vi "Mapping v10.6.4.vi"(5 "Simulate Spectra":bool, 7 "Simulate Drive":bool) -> ()   [LabVIEW 2010]
uses:
  TypeDefs/Mapping Spectra Params.ctl
  TypeDefs/Mapping Drive Params v10.6.0.ctl
  NPC3SG/TypeDefs/NPC3SG Set Positions.ctl
  NPC3SG/TypeDefs/NPC3SG Current Values.ctl
  iHR550/TypeDefs/iHR Current Values.ctl
  ITC503/TypeDefs/ITC503 Current Values.ctl
  TypeDefs/Mapping Input Parameters v10.6.2.ctl
  Symphony/TypeDefs/Symphony Area Format.ctl
  <vilib>/Utility/miscctls.llb/LVPointTypeDef.ctl
  Global Variables.vi
panel:
  in  "AutoSave Inc.":i16=20 caption="Auto Save (%)" min=10 max=160 step=1
  in  "Save Map":bool
  in  "Input Parameters":T1={"Drive Connection Port"="", "ITC503 Current Values"={"ITC503 Heater"=0.0, "ITC503 Temperature"=0.0, "ITC503 P"=0.0, "ITC503 I"=0.0, "ITC503 D"=0.0, "ITC503 Setpoint"=0.0, "ITC503 Gradient"=0.0, "ITC503 Heater Auto"=FALSE, "ITC503 PID Auto"=FALSE}, "Wavelengths (nm)"=[], "Drive Current Values"={"Drive X Position"=0.0, "Drive Y Position"=0.0, "Drive Z Position"=0.0}, "iHR Current Values"={"iHR 550 Front Entrance"=0.0, "iHR550 Side Exit"=0.0, "iHR550 Wavelength"=897.9988, "iHR550 Exit Mirror"=2, "iHR550 Grating"="1", "Grating Index"=1}, "Spectra Settings"={"Integration Time"=1.0, "Repetitions"=1, "Mapping Spectra"=TRUE}, "CCD3500 Temperature"=0.0, "Simulate Drive"=FALSE, "Simulate Spectra"=FALSE, "JYCCDLib.IJYCCDReqd"=refnum, "CCD Area"={"XStart"=1, "YStart"=1, "XStop"=2048, "YStop"=512, "XBin"=1, "YBin"=1}, "CCD Gain"=1, "CCD ADC"=0, "Drive Calibration"=path ""} {"CCD ADC" items=["20 kHz       ", " 1 MHz       ", " 1 MHz Ultra ", "500 kHz Wrap"]; "CCD Gain" items=["High Light", "Best Dynamic Range", "High Sensitivity"]; "ITC503 Current Values"."ITC503 Gradient" format="%.2f"; "ITC503 Current Values"."ITC503 Setpoint" min=-273.0 max=300000.0 step=0.0001 format="%.1f"; "ITC503 Current Values"."ITC503 I" format="%_1f"; "ITC503 Current Values"."ITC503 P" format="%_1f"; "ITC503 Current Values"."ITC503 Temperature" min=0.0 max=1645.0 step=1e-05 format="%.2f"; "ITC503 Current Values"."ITC503 Heater" min=0.0 max=100.0 step=0.01 scale=0.0..100.0; "Drive Current Values"."Drive Z Position" min=-273.0 max=300000.0 step=0.0001 format="%.3f"; "Drive Current Values"."Drive Y Position" min=-273.0 max=300000.0 step=0.0001 format="%.3f"; "Drive Current Values"."Drive X Position" min=-273.0 max=300000.0 step=0.0001 format="%.3f"; "iHR Current Values"."iHR550 Exit Mirror" items=["EntranceMirror", "ExitMirror", "Front", "Side"]; "Spectra Settings"."Repetitions" min=1 max=100 step=1; "Spectra Settings"."Integration Time" min=0.5 max=6000.0 step=1.0 format="%.1f"}
  out "JYCCDLib.IJYCCDReqd":refnum<k7>
  out "AutoClose":bool
  out "ITC503 Temperature":dbl caption="Sample (K)" min=10.0 max=160.0 step=0.1 format="%.3f"
  out "CCD3500 Temperature":dbl caption="CCD (°C)" min=10.0 max=160.0 step=0.1 format="%.1f"
  in  "CCD Current Rep.":string="0/0"
  in  "Pause":bool
  out "Current Position":T3 {"Drive Z Position" min=-273.0 max=300000.0 step=0.0001 format="%.3f"; "Drive Y Position" min=-273.0 max=300000.0 step=0.0001 format="%.3f"; "Drive X Position" min=-273.0 max=300000.0 step=0.0001 format="%.3f"}
  out "Target Position":T7={"Drive X Set"=10.0, "Drive Y Set"=10.0, "Drive Z Set"=10.0} {"Drive X Set" min=10.0 max=160.0 step=0.1 format="%.3f"; "Drive Z Set" min=10.0 max=160.0 step=0.1 format="%.3f"; "Drive Y Set" min=10.0 max=160.0 step=0.1 format="%.3f"}
  out "Progress":u8(slide) max=10 scale=0.0..100.0
  out "Objective Running":bool caption="Obj."
  out "CCD Running":bool caption="CCD"
  in  "Spectra Params":T5={"Integration Time"=10.0, "Repetitions"=10, "Mapping Spectra"=TRUE} {"Repetitions" min=1 max=100 step=1; "Integration Time" min=0.5 max=6000.0 step=1.0 format="%.1f"}
  in  "Drive Settings":refnum<visa-resource-name>
  in  "Z Position":dbl caption="Z (µm)" min=0.0 max=100.0 step=0.1 format="%.1f"
  in  "Mapping Params":T8={"X Start Position"=0.0, "X Stop Position"=10.0, "Y Start Position"=0.0, "Y Stop Position"=10.0, "Step Size"=1.0} {"Step Size" min=0.005 max=20.0 step=0.005 format="%.3f"; "Y Stop Position" min=0.0 max=140.0 step=0.005 format="%.3f"; "Y Start Position" min=0.0 max=140.0 step=0.005 format="%.3f"; "X Stop Position" min=0.0 max=140.0 step=0.005 format="%.3f"; "X Start Position" min=0.0 max=140.0 step=0.005 format="%.3f"}
  in  "Exit":bool
  out "Measuring":bool
  in  "Start":bool
  out "Filename":string
  out "Full Data":dbl[][](array[numeric])
  out "Live Data":dbl[][](array[numeric])
  in  "ITC503 Current Values":T2 {"ITC503 Gradient" format="%.2f"; "ITC503 Setpoint" min=-273.0 max=300000.0 step=0.0001 format="%.1f"; "ITC503 I" format="%_1f"; "ITC503 P" format="%_1f"; "ITC503 Temperature" min=0.0 max=1645.0 step=1e-05 format="%.2f"; "ITC503 Heater" min=0.0 max=100.0 step=0.01 scale=0.0..100.0}
  in  "iHR Current Values":T4={"iHR 550 Front Entrance"=0.0, "iHR550 Side Exit"=0.0, "iHR550 Wavelength"=897.9988, "iHR550 Exit Mirror"=2, "iHR550 Grating"="1", "Grating Index"=1} {"iHR550 Exit Mirror" items=["EntranceMirror", "ExitMirror", "Front", "Side"]}
  in  "Wavelengths (nm)":dbl[](array[numeric])
  # "Mapping"
  # "Status"
  # "Active"
  # "Target"
  # "Current"
  # "Spectral"
  # "Spectral / Video Mapping"
  # "Drive Settings"
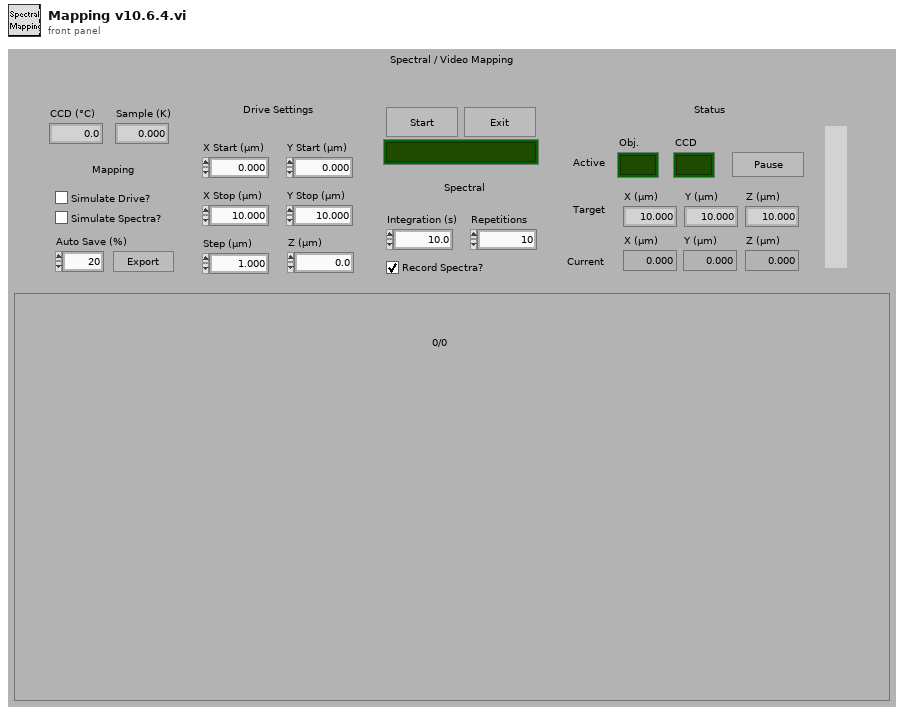
[diagram p1: front panel]
types:
  T1 = typedef "Mapping Input Parameters v10.6.2.ctl" = cluster{"Drive Connection Port":refnum<visa-resource-name>, "ITC503 Current Values":T2, "Wavelengths (nm)":dbl[], "Drive Current Values":T3, "iHR Current Values":T4, "Spectra Settings":T5, "CCD3500 Temperature":dbl, "Simulate Drive":bool, "Simulate Spectra":bool, "JYCCDLib.IJYCCDReqd":refnum<k7>, "CCD Area":T6, "CCD Gain":u16, "CCD ADC":u16, "Drive Calibration":path}
  T2 = typedef "ITC503 Current Values.ctl" = cluster{"ITC503 Heater":dbl, "ITC503 Temperature":dbl, "ITC503 P":dbl, "ITC503 I":dbl, "ITC503 D":dbl, "ITC503 Setpoint":dbl, "ITC503 Gradient":dbl, "ITC503 Heater Auto":bool, "ITC503 PID Auto":bool}
  T3 = typedef "NPC3SG Current Values.ctl" = cluster{"Drive X Position":dbl, "Drive Y Position":dbl, "Drive Z Position":dbl}
  T4 = typedef "iHR Current Values.ctl" = cluster{"iHR 550 Front Entrance":dbl, "iHR550 Side Exit":dbl, "iHR550 Wavelength":dbl, "iHR550 Exit Mirror":i32, "iHR550 Grating":string, "Grating Index":i32}
  T5 = typedef "Mapping Spectra Params.ctl" = cluster{"Integration Time":dbl, "Repetitions":u16, "Mapping Spectra":bool}
  T6 = typedef "Symphony Area Format.ctl" = cluster{"XStart":i32, "YStart":i32, "XStop":i32, "YStop":i32, "XBin":i32, "YBin":i32}
  T7 = typedef "NPC3SG Set Positions.ctl" = cluster{"Drive X Set":dbl, "Drive Y Set":dbl, "Drive Z Set":dbl}
  T8 = typedef "Mapping Drive Params v10.6.0.ctl" = cluster{"X Start Position":dbl, "X Stop Position":dbl, "Y Start Position":dbl, "Y Stop Position":dbl, "Step Size":dbl}
  T9 = typedef "LVPointTypeDef.ctl" = cluster{"Horizontal":i16, "Vertical":i16}
  T10 = cluster{"Intensities":dbl[], "Wavelengths":dbl[]}[]
  T11 = cluster{"Intensities":dbl[], "Wavelengths":dbl[]}
  T12 = enum32{"invalid app kind", "Development System", "Run Time System", "Student Edition", "Embedded LabVIEW", "Evaluation", "Custom"}
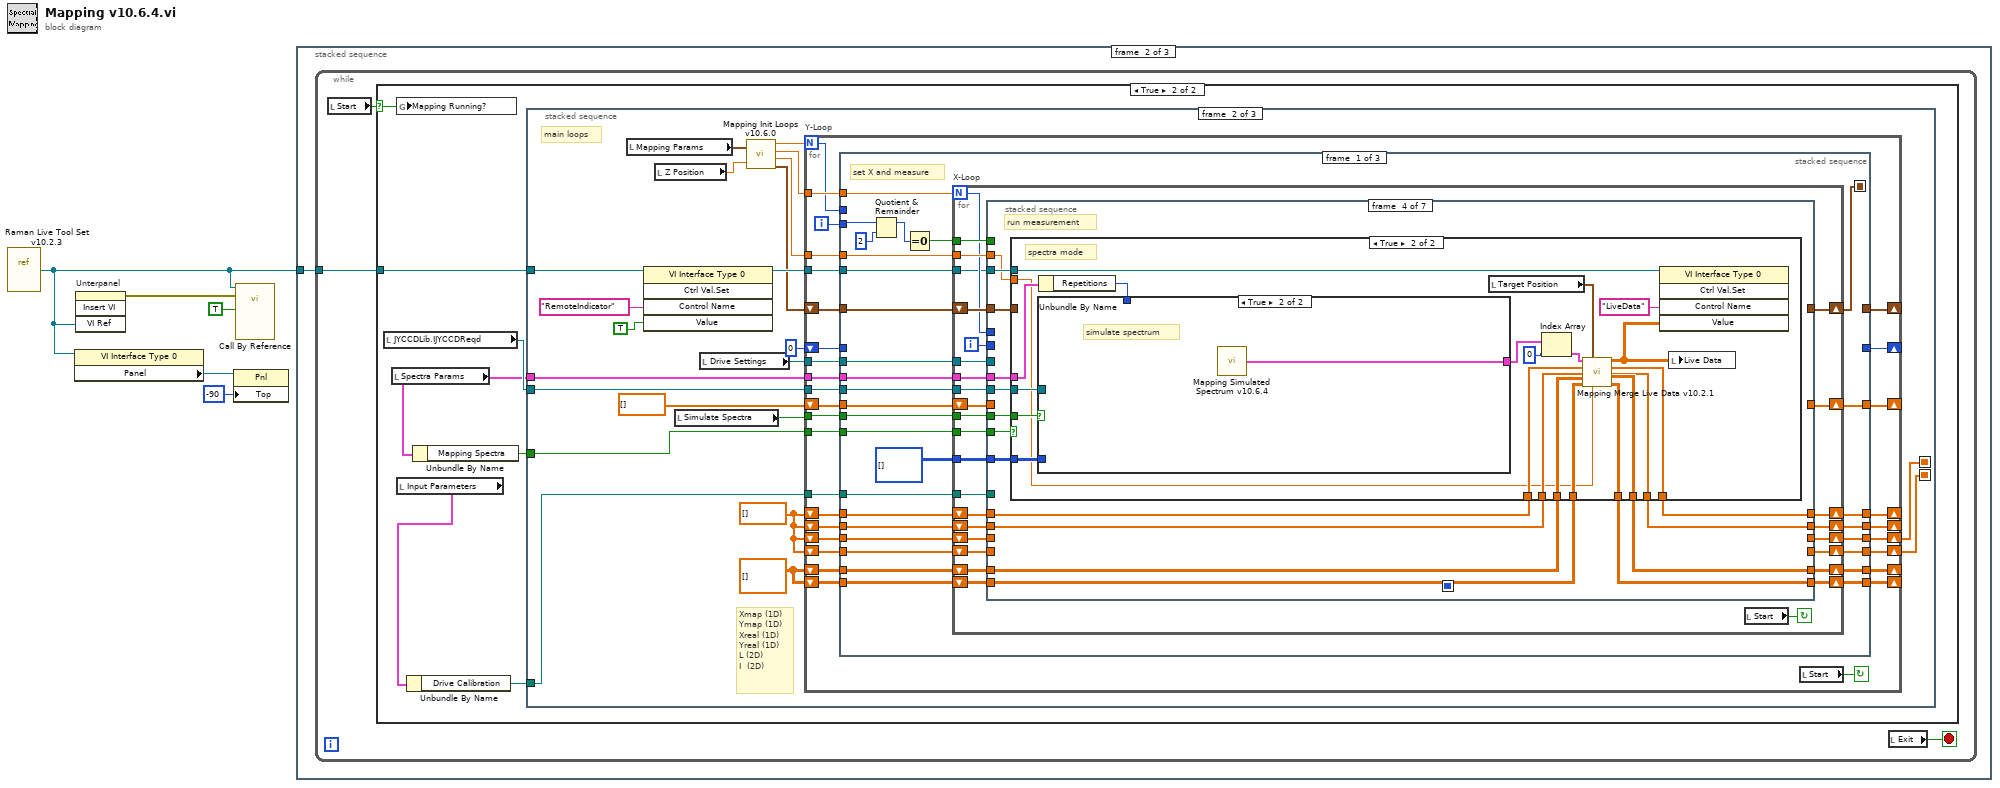
[diagram p0: block diagram]
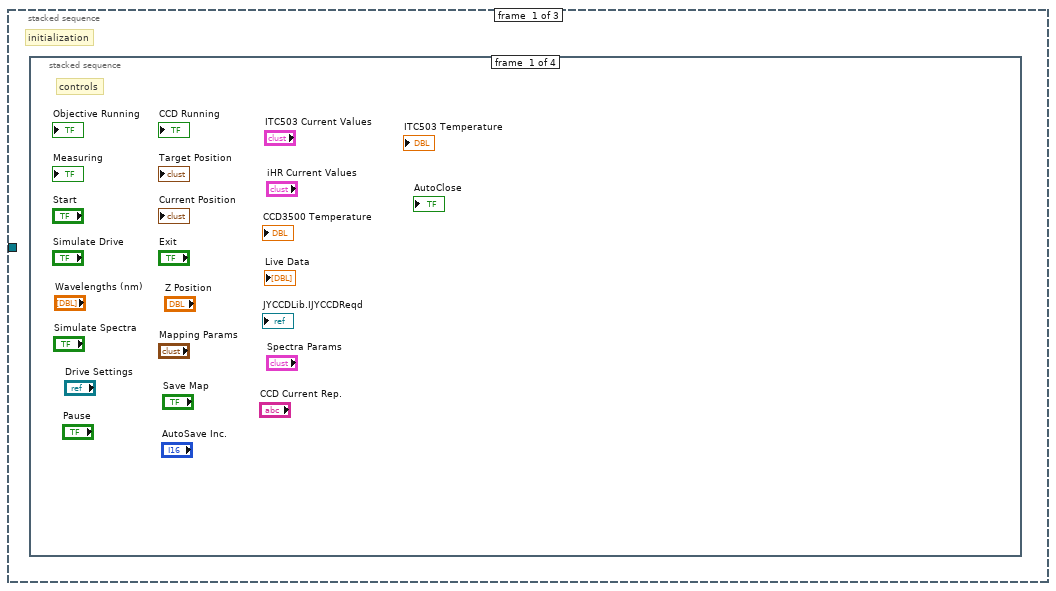
[diagram p2: hidden frame]
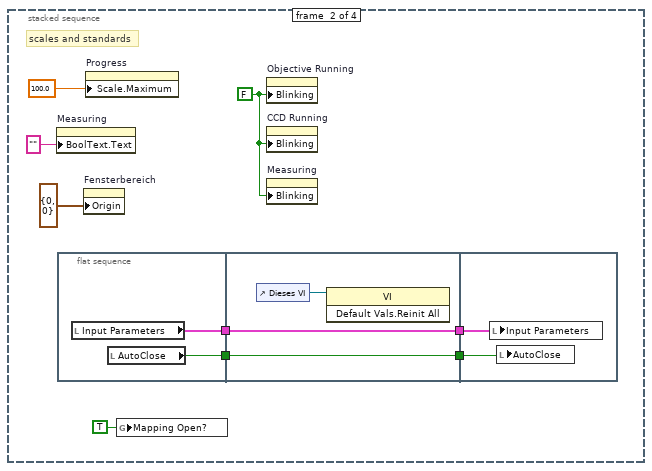
[diagram p3: hidden frame]
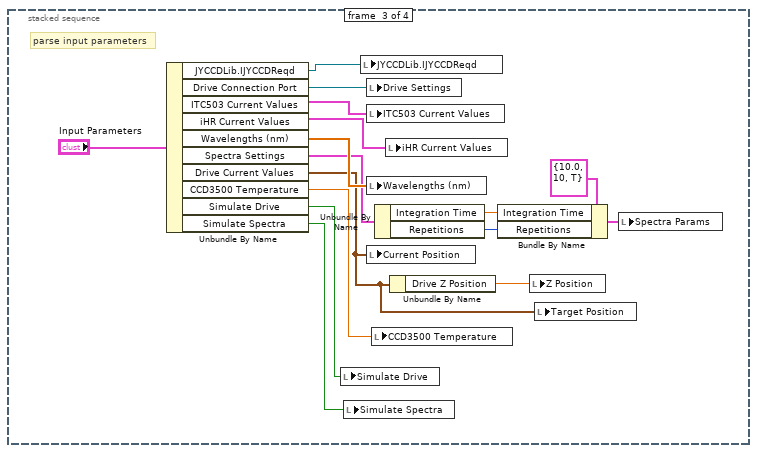
[diagram p4: hidden frame]
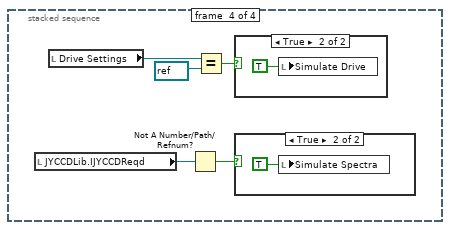
[diagram p5: hidden frame]
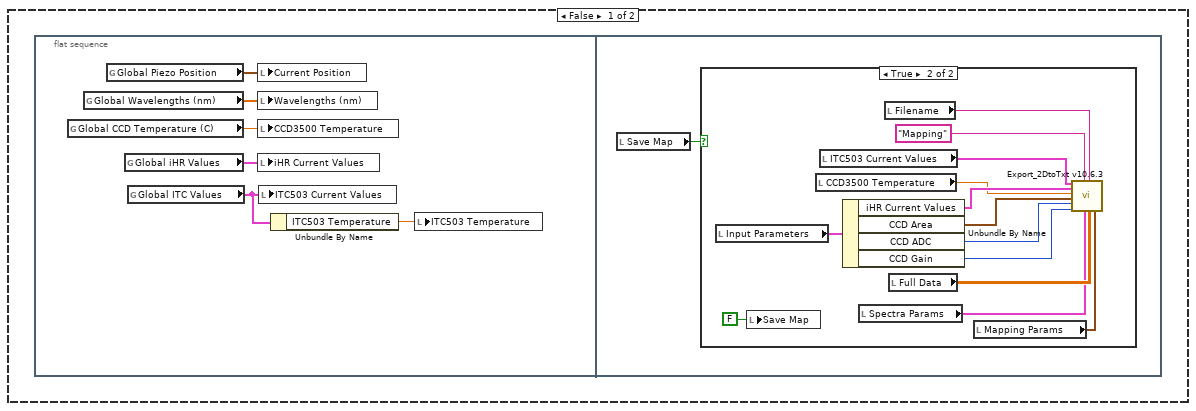
[diagram p8: hidden frame]
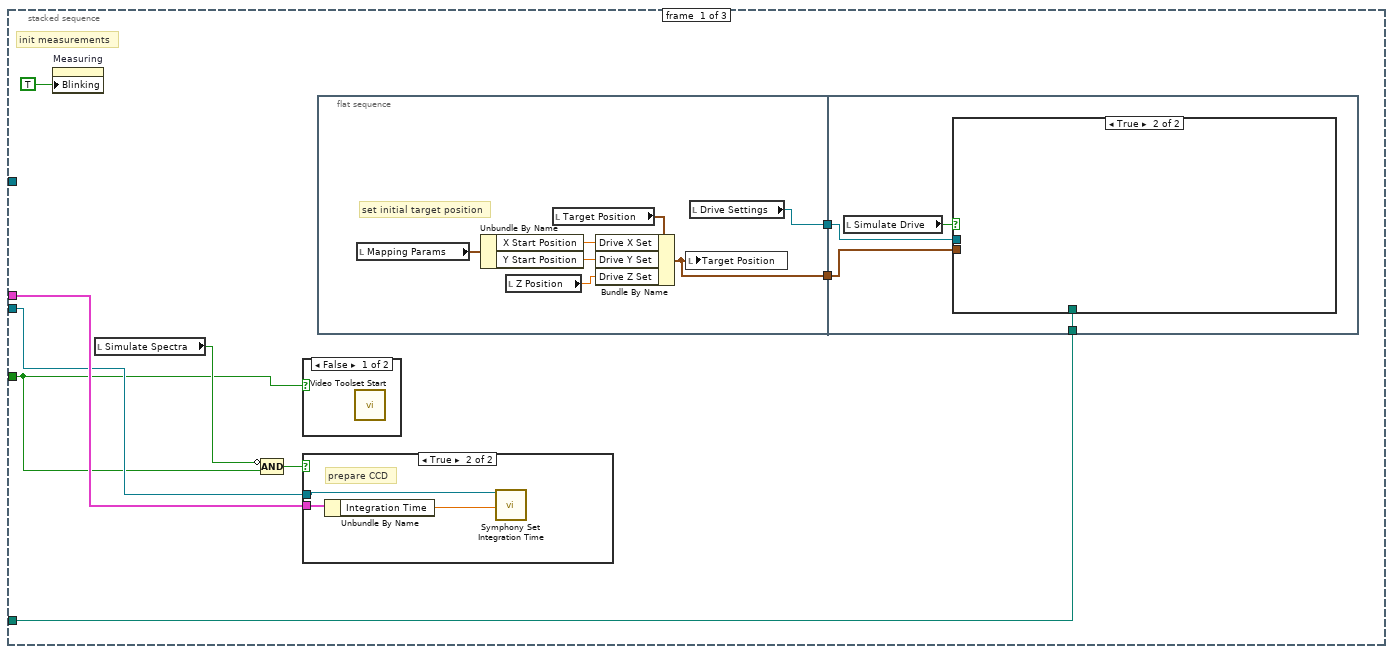
[diagram p10: hidden frame]
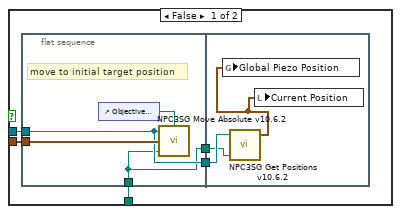
[diagram p13: hidden frame]
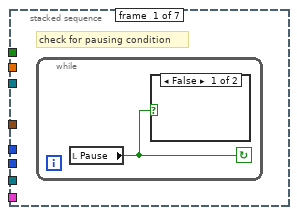
[diagram p14: hidden frame]
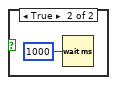
[diagram p15: hidden frame]
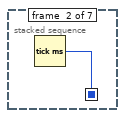
[diagram p16: hidden frame]
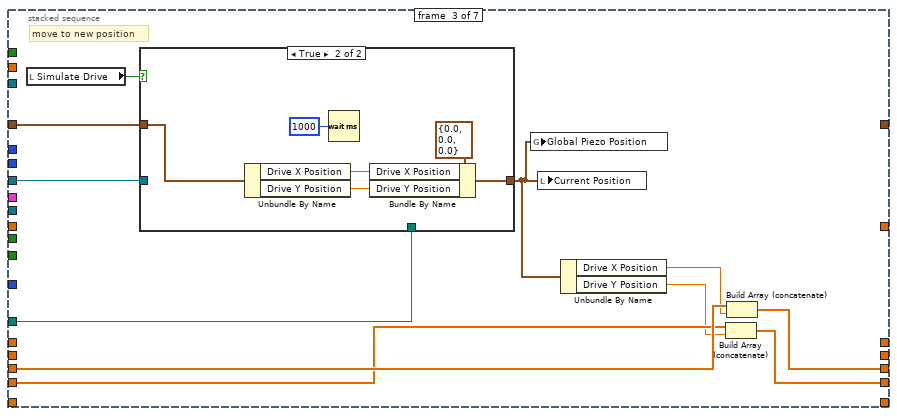
[diagram p17: hidden frame]
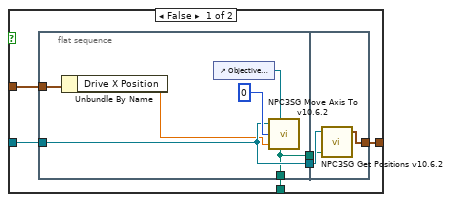
[diagram p18: hidden frame]
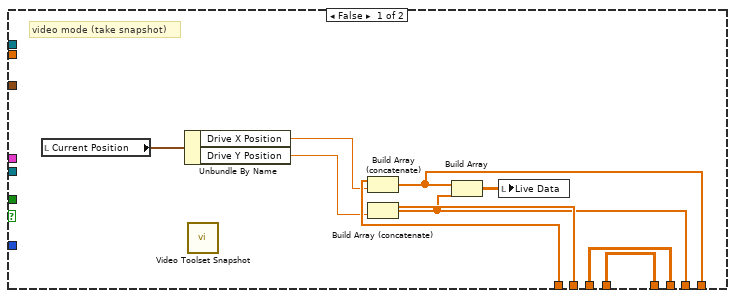
[diagram p19: hidden frame]
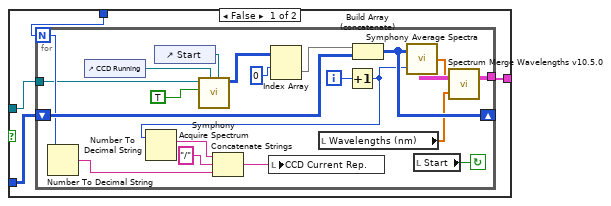
[diagram p20: hidden frame]
diagram:
  n1 = vi-ref "Raman Live Tool Set v10.2.3.vi"() -> (w3:refnum<vi>)
  n2 = property class="VI Interface Type 0"(reference=w3) -> ("Panel"=w2:refnum<vi>)  [unwired: 1 in, 2 out]
  n3 = invoke on="Unterpanel" class="Unterpanel" method="Insert VI"("VI Ref"=w3) -> (error out=w5:errorcluster)  [unwired: 3 in, 3 out]
  n4 = property class="Pnl"(reference=w2, "Top"=-90 ("Position:Oben")) -> ()  [unwired: 1 in, 2 out]
  n5 = call-by-ref "?"(reference=w3, error in=w5, "RemoteIndicator"=TRUE) -> ()  [unwired: 3 in, 2 out]
  n6 = stacked-sequence {
    tunnel: w3 -> [_ w45 w472]
    frame #0 {
      # "initialization"
      n7 = stacked-sequence {
        frame #0 {
          # "controls"
        }
        frame #1 {
          w12 = FALSE ("Blinkend")
          # "scales and standards"
          n8 = property on="Measuring" class="Bool (strict)"("BoolText.Text"="" ("Boolescher Text.Text")) -> ()  [unwired: 2 in, 2 out]
          n9 = flat-sequence {
            tunnel: [w16] -> w9
            tunnel: [w15] -> w6
            tunnel: [w18] -> w10
            tunnel: w9 -> [w18]
            tunnel: [w17] -> w7
            tunnel: w6 -> [w17]
            tunnel: w10 -> [w21]
            tunnel: w7 -> [w20]
            frame #0 {
              n10 = local read "Input Parameters"() -> (w16:T1)
              n11 = local read "AutoClose"() -> (w15:bool)
            }
            frame #1 {
              n12 = control-ref of="Dieses VI"() -> (w19:refnum<vi>)
              n13 = invoke class="VI" method="Default Vals.Reinit All"(reference=w19) -> ()  [unwired: 2 in, 3 out]
            }
            frame #2 {
              n14 = local write "Input Parameters"(w21) -> ()
              n15 = local write "AutoClose"(w20) -> ()
            }
          }
          n16 = property on="Fensterbereich" class="Pane"("Origin"=T9 {"Horizontal"=0, "Vertical"=0}) -> ()  [unwired: 2 in, 2 out]
          n17 = property on="Progress" class="Slide (strict)"("Scale.Maximum"=100.0 ("Skalierung.Bereich:Maximum")) -> ()  [unwired: 2 in, 2 out]
          n18 = global write "Global Variables.vi" "Mapping Open?"(TRUE ("Mapping Open?")) -> ()
          n19 = property on="Objective Running" class="Bool (strict)"("Blinking"=w12) -> ()  [unwired: 2 in, 2 out]
          n20 = property on="CCD Running" class="Bool (strict)"("Blinking"=w12) -> ()  [unwired: 2 in, 2 out]
          n21 = property on="Measuring" class="Bool (strict)"("Blinking"=w12) -> ()  [unwired: 2 in, 2 out]
        }
        frame #2 {
          # "parse input parameters"
          n22 = Unbundle By Name("Input Parameters") -> ("JYCCDLib.IJYCCDReqd"=w25:refnum<k7>, "Drive Connection Port"=w22:refnum<visa-resource-name>, "ITC503 Current Values"=w37:T2, "iHR Current Values"=w28:T4, "Wavelengths (nm)"=w36:dbl[], "Spectra Settings"=w34:T5, "Drive Current Values"=w23:T3, "CCD3500 Temperature"=w29:dbl, "Simulate Drive"=w27:bool, "Simulate Spectra"=w26:bool)
          n23 = local write "Simulate Drive"(w27) -> ()
          n24 = local write "Simulate Spectra"(w26) -> ()
          n25 = local write "JYCCDLib.IJYCCDReqd"(w25) -> ()
          n26 = local write "Drive Settings"(w22) -> ()
          n27 = local write "ITC503 Current Values"(w37) -> ()
          n28 = local write "Wavelengths (nm)"(w36) -> ()
          n29 = local write "Current Position"(w23) -> ()
          n30 = local write "CCD3500 Temperature"(w29) -> ()
          n31 = Unbundle By Name(w34) -> ("Integration Time"=w32:dbl, "Repetitions"=w31:u16)
          n32 = local write "iHR Current Values"(w28) -> ()
          n33 = Unbundle By Name(w23) -> ("Drive Z Position"=w35:dbl)
          n34 = Bundle By Name(cluster=T5 {"Integration Time"=10.0, "Repetitions"=10, "Mapping Spectra"=TRUE} ("Mapping Spectra Settings"), "Integration Time"=w32, "Repetitions"=w31) -> (w30:T5)
          n35 = local write "Z Position"(w35) -> ()
          n36 = local write "Target Position"(w23) -> ()
          n37 = local write "Spectra Params"(w30) -> ()
        }
        frame #3 {
          n38 = local read "JYCCDLib.IJYCCDReqd"() -> (w39:refnum<k7>)
          n39 = local read "Drive Settings"() -> (w40:refnum<visa-resource-name>)
          n40 = Not A Number/Path/Refnum?(number/path/refnum=w39) -> (NaN/Path/Refnum?=w38:bool)
          n41 = Equal?(x=w40, y=refnum<visa-resource-name> refnum ("Drive Settings")) -> (x = y?=w41:bool)
          n42 = case shown="True" w41 {
            frame False {
            }
            frame True {
              n43 = local write "Simulate Drive"(TRUE ("Simulate Drive")) -> ()
            }
          }
          n44 = case shown="True" w38 {
            frame False {
            }
            frame True {
              n45 = local write "Simulate Spectra"(TRUE ("Simulate Drive")) -> ()
            }
          }
        }
      }
    }
    frame #1 {
      n46 = while {
        tunnel: w45 -> [w48]
        stop <- w47 stop-if-true
        n47 = local read "Start"() -> (w46:bool)
        n48 = case shown="True" w46 {
          selector: w46 -> [_ w72]
          tunnel: w48 -> [_ w75]
          frame False {
            n49 = flat-sequence {
              frame #0 {
                n50 = global read "Global Variables.vi" "Global CCD Temperature (C)"() -> (w54:dbl)
                n51 = global read "Global Variables.vi" "Global Wavelengths (nm)"() -> (w52:dbl[])
                n52 = global read "Global Variables.vi" "Global Piezo Position"() -> (w53:T3)
                n53 = global read "Global Variables.vi" "Global iHR Values"() -> (w51:T4)
                n54 = global read "Global Variables.vi" "Global ITC Values"() -> (w50:T2)
                n55 = local write "Current Position"(w53) -> ()
                n56 = local write "Wavelengths (nm)"(w52) -> ()
                n57 = local write "CCD3500 Temperature"(w54) -> ()
                n58 = local write "iHR Current Values"(w51) -> ()
                n59 = local write "ITC503 Current Values"(w50) -> ()
                n60 = Unbundle By Name(w50) -> ("ITC503 Temperature"=w49:dbl)
                n61 = local write "ITC503 Temperature"(w49) -> ()
              }
              frame #1 {
                n62 = local read "Save Map"() -> (w55:bool)
                n63 = case shown="True" w55 {
                  frame False {
                  }
                  frame True {
                    n64 = local read "Input Parameters"() -> (w64:T1)
                    n65 = local write "Save Map"(FALSE ("Save Map")) -> ()
                    n66 = local read "CCD3500 Temperature"() -> (w58:dbl)
                    n67 = local read "ITC503 Current Values"() -> (w61:T2)
                    n68 = Unbundle By Name(w64) -> ("iHR Current Values"=w59:T4, "CCD Area"=w60:T6, "CCD ADC"=w63:u16, "CCD Gain"=w62:u16)
                    n69 = local read "Spectra Params"() -> (w57:T5)
                    n70 = local read "Filename"() -> (w67:string)
                    n71 = local read "Full Data"() -> (w65:dbl[][])
                    n72 = local read "Mapping Params"() -> (w56:T8)
                    n73 = call "Export_2DtoTxt v10.6.3.vi"("ITC503 Current Values"=w61, "iHR Current Values"=w59, "CCD Temperature"=w58, "CCD Area"=w60, "CCD ADC"=w63, "CCD Gain"=w62, "Export Type"="Mapping", "Spectra Settings"=w57, "Filename"=w67, "Data (2D)"=w65, "Mapping Parameters"=w56) -> ()  [unwired: 8 in, 1 out]
                  }
                }
              }
            }
          }
          frame True {
            n74 = local read "JYCCDLib.IJYCCDReqd"() -> (w74:refnum<k7>)
            n75 = local read "Spectra Params"() -> (w73:T5)
            n76 = global write "Global Variables.vi" "Mapping Running?"(w72) -> ()
            n77 = local read "Input Parameters"() -> (w70:T1)
            n78 = Unbundle By Name(w70) -> ("Drive Calibration"=w69:path)
            n79 = Unbundle By Name(w73) -> ("Mapping Spectra"=w71:bool)
            n80 = stacked-sequence {
              seq-local: [_ w113 _] -> [_ _ w447]
              seq-local: [_ w114 _] -> [_ _ w446]
              tunnel: w75 -> [_ w124 _]
              tunnel: w71 -> [w77 w123 w448]
              tunnel: w73 -> [w79 w121 _]
              tunnel: w74 -> [w78 w120 _]
              tunnel: w69 -> [w76 w112 _]
              frame #0 {
                # "init measurements"
                n81 = property on="Measuring" class="Bool (strict)"("Blinking"=TRUE ("Blinkend")) -> ()  [unwired: 2 in, 2 out]
                n82 = local read "Simulate Spectra"() -> (w81:bool)
                n83 = Compound Arithmetic op=AND(invert w81, w77) -> (w80:bool)
                n84 = case shown="False" w77 {
                  frame False {
                    n85 = call "Video Toolset Start.vi"() -> ()  [unwired: 3 in]
                  }
                  frame True {
                  }
                }
                n86 = case shown="True" w80 {
                  tunnel: w78 -> [_ w87]
                  tunnel: w79 -> [_ w86]
                  frame False {
                  }
                  frame True {
                    # "prepare CCD"
                    n87 = Unbundle By Name(w86) -> ("Integration Time"=w85:dbl)
                    n88 = call "Symphony Set Integration Time.vi"("JYCCDLib.IJYCCDReqd"=w87, "Integration (s)"=w85) -> ()  [unwired: 13 in, 1 out]
                  }
                }
                n89 = flat-sequence {
                  tunnel: [w89] -> w83
                  tunnel: [w88] -> w82
                  tunnel: w83 -> [w96]
                  tunnel: w82 -> [w97]
                  tunnel: w76 -> [w95]
                  frame #0 {
                    # "set initial target position"
                    n90 = local read "Mapping Params"() -> (w94:T8)
                    n91 = Unbundle By Name(w94) -> ("X Start Position"=w92:dbl, "Y Start Position"=w91:dbl)
                    n92 = local read "Z Position"() -> (w90:dbl)
                    n93 = local read "Target Position"() -> (w93:T7)
                    n94 = Bundle By Name(cluster=w93, "Drive X Set"=w92, "Drive Y Set"=w91, "Drive Z Set"=w90) -> (w89:T7)
                    n95 = local write "Target Position"(w89) -> ()
                    n96 = local read "Drive Settings"() -> (w88:refnum<visa-resource-name>)
                  }
                  frame #1 {
                    n97 = local read "Simulate Drive"() -> (w98:bool)
                    n98 = case shown="True" w98 {
                      tunnel: w97 -> [w103 _]
                      tunnel: w96 -> [w101 _]
                      tunnel: w95 -> [w100 _]
                      frame False {
                        n99 = flat-sequence {
                          tunnel: w103 -> [w105]
                          tunnel: [w105] -> w102
                          tunnel: w101 -> [w106]
                          tunnel: w100 -> [w104]
                          tunnel: [w104] -> w99
                          tunnel: w102 -> [w109]
                          tunnel: w99 -> [w108]
                          frame #0 {
                            # "move to initial target position"
                            n100 = control-ref of="Objective Running"() -> (w107:refnum<vi>)
                            n101 = call "NPC3SG Move Absolute v10.6.2.vi"("Running"=w107, "Calibration File"=w104, "Drive New Abs. Positions"=w106, "Drive Visa Name"=w105) -> ()  [unwired: 1 in]
                          }
                          frame #1 {
                            n102 = call "NPC3SG Get Positions v10.6.2.vi"("Drive Visa Name"=w109, "Calibration File"=w108) -> ("Drive Current Values"=w110:T3)  [unwired: 5 in]
                            n103 = global write "Global Variables.vi" "Global Piezo Position"(w110) -> ()
                            n104 = local write "Current Position"(w110) -> ()
                          }
                        }
                      }
                      frame True {
                      }
                    }
                  }
                }
              }
              frame #1 {
                w132 = dbl[][] []
                w115 = dbl[] []
                # "main loops"
                # "Xmap (1D)\nYmap (1D)\nXreal (1D)\nYreal (1D)\nL (2D)\nI  (2D)"
                n105 = local read "Mapping Params"() -> (w118:T8)
                n106 = invoke class="VI Interface Type 0" method="Ctrl Val.Set"(reference=w124, "Control Name"="RemoteIndicator" ("Elementname"), "Value"=TRUE) -> (reference out=w126:refnum<vi>)  [unwired: 2 in, 4 out]
                n107 = local read "Z Position"() -> (w117:dbl)
                n108 = local read "Simulate Spectra"() -> (w116:bool)
                n109 = local read "Drive Settings"() -> (w119:refnum<visa-resource-name>)
                n110 = call "Mapping Init Loops v10.6.0.vi"("Z Position"=w117, "Mapping Params"=w118) -> ("Start Positions"=w125:T3, "Step Size"=w127:dbl, "X Steps"=w128:dbl, "Y Steps"=w129:dbl)
                n111 = for "Y-Loop" {
                  N: w129 -> [w148]
                  tunnel: w128 -> [w161]
                  tunnel: w127 -> [w160]
                  shift-right: [w146] -> _
                  shift-left: w125 -> [w147]
                  shift-right: [w152] -> _
                  shift-left: w132 -> [w156]
                  shift-right: [w153] -> _
                  shift-left: w132 -> [w157]
                  shift-right: [w155] -> _
                  shift-left: w115 -> [w159]
                  shift-right: [w154] -> _
                  shift-left: w115 -> [w158]
                  tunnel: w126 -> [w150]
                  tunnel: w116 -> [w149]
                  tunnel: w119 -> [w145]
                  tunnel: w123 -> [w144]
                  tunnel: w121 -> [w143]
                  shift-right: [w141] -> _
                  shift-left: dbl[] [] -> [w142]
                  tunnel: w120 -> [w140]
                  shift-right: [w137] -> w114
                  shift-left: w115 -> [w138]
                  shift-right: [w136] -> w113
                  shift-left: w115 -> [w139]
                  tunnel: w112 -> [w135]
                  shift-right: [w134] -> _
                  shift-left: i16 0 ("Progress") -> [w133]
                  i -> [w151]
                  stop <- w162 continue-if-true
                  n112 = stacked-sequence {
                    seq-local: [w177 _ _] -> [_ _ w417]
                    tunnel: w161 -> [w192 _ _]
                    tunnel: w160 -> [w191 _ w418]
                    tunnel: w159 -> [w190 _ _]
                    tunnel: w158 -> [w189 _ _]
                    tunnel: w157 -> [w188 _ _]
                    tunnel: w156 -> [w164 _ _]
                    tunnel: [w187 _ _] -> w155
                    tunnel: [w186 _ _] -> w154
                    tunnel: [w185 _ _] -> w153
                    tunnel: [w184 _ _] -> w152
                    tunnel: w151 -> [w181 _ w421]
                    tunnel: w150 -> [w179 _ _]
                    tunnel: w149 -> [w178 _ _]
                    tunnel: w148 -> [_ _ w419]
                    tunnel: w147 -> [w176 _ _]
                    tunnel: [_ _ w415] -> w146
                    tunnel: w145 -> [w175 _ w416]
                    tunnel: w144 -> [w174 _ _]
                    tunnel: w143 -> [w173 _ _]
                    tunnel: w142 -> [w172 _ _]
                    tunnel: [w171 _ _] -> w141
                    tunnel: w140 -> [w170 _ _]
                    tunnel: w139 -> [w168 w383 _]
                    tunnel: w138 -> [w167 w382 _]
                    tunnel: [w166 _ _] -> w137
                    tunnel: [w165 _ _] -> w136
                    tunnel: w135 -> [w163 _ w409]
                    tunnel: [_ w381 _] -> w134
                    tunnel: w133 -> [_ w380 _]
                    frame #0 {
                      # "set X and measure"
                      n113 = Quotient & Remainder(x=w181, y=2) -> (x-y*floor(x/y)=w182:i32)  [unwired: 1 out]
                      n114 = Equal To 0?(x=w182) -> (x = 0?=w180:bool)
                      n115 = for "X-Loop" {
                        N: w192 -> [w207]
                        tunnel: w191 -> [w219]
                        shift-right: [w218] -> w177
                        shift-left: w176 -> [w220]
                        shift-right: [w213] -> w187
                        shift-left: w190 -> [w217]
                        shift-right: [w212] -> w186
                        shift-left: w189 -> [w216]
                        shift-right: [w210] -> w185
                        shift-left: w188 -> [w215]
                        shift-right: [w211] -> w184
                        shift-left: w164 -> [w214]
                        tunnel: w180 -> [w209]
                        tunnel: w179 -> [w206]
                        tunnel: w178 -> [w205]
                        tunnel: w175 -> [w204]
                        tunnel: w174 -> [w203]
                        tunnel: w173 -> [w202]
                        shift-right: [w201] -> w171
                        shift-left: w172 -> [w200]
                        tunnel: w170 -> [w199]
                        tunnel: u16[][] [] -> [w198]
                        shift-right: [w194] -> w165
                        shift-left: w168 -> [w197]
                        shift-right: [w195] -> w166
                        shift-left: w167 -> [w196]
                        tunnel: w163 -> [w193]
                        i -> [w208]
                        stop <- w221 continue-if-true
                        n116 = stacked-sequence {
                          seq-local: [_ w224 _ _ _ _ _] -> [_ _ _ _ _ w359 _]
                          tunnel: w220 -> [_ _ w235 w272 w336 _ _]
                          tunnel: w219 -> [_ _ _ w257 w334 _ _]
                          tunnel: [_ _ _ _ w333 _ _] -> w218
                          tunnel: w217 -> [_ _ _ w271 _ _ _]
                          tunnel: w216 -> [_ _ _ w270 _ _ _]
                          tunnel: w215 -> [_ _ _ w268 _ _ _]
                          tunnel: w214 -> [_ _ _ w269 _ _ w368]
                          tunnel: [_ _ _ w267 _ _ _] -> w213
                          tunnel: [_ _ _ w266 _ _ _] -> w212
                          tunnel: [_ _ _ w265 _ _ _] -> w211
                          tunnel: [_ _ _ w264 _ _ _] -> w210
                          tunnel: w209 -> [_ _ _ _ w335 _ _]
                          tunnel: w208 -> [_ _ _ _ w339 _ _]
                          tunnel: w207 -> [_ _ _ _ w337 _ _]
                          tunnel: w206 -> [_ _ _ w263 _ _ _]
                          tunnel: w205 -> [_ _ _ w262 _ _ _]
                          tunnel: w204 -> [_ _ w233 _ _ _ _]
                          tunnel: w203 -> [_ _ _ w261 _ _ _]
                          tunnel: w202 -> [_ _ _ w259 _ _ w370]
                          tunnel: [_ _ _ _ _ w356 _] -> w201
                          tunnel: w200 -> [_ _ _ _ _ w358 w369]
                          tunnel: w199 -> [_ _ _ w260 _ _ _]
                          tunnel: w198 -> [_ _ _ w258 _ _ _]
                          tunnel: w197 -> [_ _ w232 _ _ _ _]
                          tunnel: w196 -> [_ _ w231 _ _ _ _]
                          tunnel: [_ _ w228 _ _ _ _] -> w195
                          tunnel: [_ _ w227 _ _ _ _] -> w194
                          tunnel: w193 -> [_ _ w225 _ _ _ _]
                          frame #0 {
                            # "check for pausing condition"
                            n117 = while {
                              stop <- w222 continue-if-true
                              n118 = local read "Pause"() -> (w222:bool)
                              n119 = case shown="False" w222 {
                                frame False {
                                }
                                frame True {
                                n120 = Wait (ms)(milliseconds to wait=u32 1000) -> ()  [unwired: 1 out]
                                }
                              }
                            }
                          }
                          frame #1 {
                            n121 = Tick Count (ms)() -> (millisecond timer value=w224:u32)
                          }
                          frame #2 {
                            # "move to new position"
                            n122 = local read "Simulate Drive"() -> (w234:bool)
                            n123 = case shown="True" w234 {
                              tunnel: w235 -> [w241 w255]
                              tunnel: w233 -> [w240 _]
                              tunnel: [w238 w251] -> w226
                              tunnel: w225 -> [w237 _]
                              frame False {
                                n124 = flat-sequence {
                                tunnel: w241 -> [w244]
                                tunnel: w240 -> [w245]
                                tunnel: [w245] -> w239
                                tunnel: w237 -> [w242]
                                tunnel: [w242] -> w236
                                tunnel: w239 -> [w250]
                                tunnel: [w249] -> w238
                                tunnel: w236 -> [w248]
                                frame #0 {
                                n125 = Unbundle By Name(w244) -> ("Drive X Position"=w243:dbl)
                                n126 = control-ref of="Objective Running"() -> (w246:refnum<vi>)
                                n127 = call "NPC3SG Move Axis To v10.6.2.vi"("Drive Visa Name"=w245, "Running"=w246, "Axis"=0, "Drive Set"=w243, "Calibration File"=w242) -> ()  [unwired: 2 in, 1 out]
                                }
                                frame #1 {
                                n128 = call "NPC3SG Get Positions v10.6.2.vi"("Drive Visa Name"=w250, "Calibration File"=w248) -> ("Drive Current Values"=w249:T3)  [unwired: 5 in]
                                }
                                }
                              }
                              frame True {
                                n129 = Unbundle By Name(w255) -> ("Drive X Position"=w256:dbl, "Drive Y Position"=w253:dbl)
                                n130 = Wait (ms)(milliseconds to wait=u32 1000 ("Zu wartende ms")) -> ()  [unwired: 1 out]
                                n131 = Bundle By Name(cluster=T3 {"Drive X Position"=0.0, "Drive Y Position"=0.0, "Drive Z Position"=0.0} ("Drive Current Values"), "Drive X Position"=w256, "Drive Y Position"=w253) -> (w251:T3)
                              }
                            }
                            n132 = global write "Global Variables.vi" "Global Piezo Position"(w226) -> ()
                            n133 = local write "Current Position"(w226) -> ()
                            n134 = Unbundle By Name(w226) -> ("Drive X Position"=w230:dbl, "Drive Y Position"=w229:dbl)
                            n135 = Build Array (concatenate)(w231, w229) -> (w228:dbl[])
                            n136 = Build Array (concatenate)(w232, w230) -> (w227:dbl[])
                          }
                          frame #3 {
                            # "run measurement"
                            n137 = case shown="True" w261 {
                              tunnel: w272 -> [_ _]
                              tunnel: w271 -> [w279 w300]
                              tunnel: w270 -> [w278 w299]
                              tunnel: w269 -> [w281 w297]
                              tunnel: w268 -> [w282 w298]
                              tunnel: [w276 w294] -> w267
                              tunnel: [w277 w293] -> w266
                              tunnel: [w281 w296] -> w265
                              tunnel: [w282 w295] -> w264
                              tunnel: w263 -> [_ w302]
                              tunnel: w262 -> [_ w301]
                              tunnel: w260 -> [_ w290]
                              tunnel: w259 -> [_ w289]
                              tunnel: w258 -> [_ w287]
                              tunnel: w257 -> [_ w283]
                              frame False {
                                # "video mode (take snapshot)"
                                n138 = local read "Current Position"() -> (w280:T3)
                                n139 = Unbundle By Name(w280) -> ("Drive X Position"=w275:dbl, "Drive Y Position"=w274:dbl)
                                n140 = call "Video Toolset Snapshot.vi"() -> ()  [unwired: 12 in]
                                n141 = Build Array (concatenate)(w279, w275) -> (w276:dbl[])
                                n142 = Build Array (concatenate)(w278, w274) -> (w277:dbl[])
                                n143 = Build Array(w276, w277) -> (w273:dbl[][])
                                n144 = local write "Live Data"(w273) -> ()
                              }
                              frame True {
                                # "spectra mode"
                                n145 = Unbundle By Name(w289) -> ("Repetitions"=w288:u16)
                                n146 = case shown="True" w301 {
                                tunnel: [w306 w328] -> w286
                                tunnel: w290 -> [w307 _]
                                tunnel: w288 -> [w305 _]
                                tunnel: w287 -> [w304 _]
                                frame False {
                                n147 = for {
                                N: w305 -> [w314]
                                shift-right: [w325] -> _
                                shift-left: w304 -> [w326]
                                tunnel: [w323] -> w306
                                tunnel: w307 -> [w312]
                                i -> [w327]
                                stop <- w321 continue-if-true
                                n148 = Number To Decimal String(number=w314) -> (decimal integer string=w317:string)  [unwired: 1 in]
                                n149 = control-ref of="CCD Running"() -> (w320:refnum<vi>)
                                n150 = control-ref of="Start"() -> (w319:refnum<vi>)
                                n151 = call "Symphony Acquire Spectrum.vi"("Acquire"=w319, "Running"=w320, "ShutterOpen"=TRUE, "JYCCDLib.IJYCCDReqd"=w312) -> ("Raw Data"=w309:i32[][])  [unwired: 6 in, 1 out]
                                n152 = Index Array(array=w309, index (row)=0) -> (element=w308:i32[])  [unwired: 1 in]
                                n153 = local read "Wavelengths (nm)"() -> (w322:dbl[])
                                n154 = Increment(x=w327) -> (x+1=w313:i32)
                                n155 = Number To Decimal String(number=w313) -> (decimal integer string=w316:string)  [unwired: 1 in]
                                n156 = Concatenate Strings(w316, "/" ("string"), w317) -> (w315:string)
                                n157 = local write "CCD Current Rep."(w315) -> ()
                                n158 = Build Array (concatenate)(w308, w326) -> (w325:i32[][])
                                n159 = call "Symphony Average Spectra.vi"("Repetitions"=w313, "Raw Spectra"=w325) -> ("Raw Spectrum"=w324:dbl[])
                                n160 = local read "Start"() -> (w321:bool)
                                n161 = call "Spectrum Merge Wavelengths v10.5.0.vi"("Wavelengths (nm)"=w322, "Raw Spectrum"=w324) -> ("Spectrum-Cluster"=w323:T10)  [unwired: 1 out]
                                }
                                }
                                frame True {
                                # "simulate spectrum"
                                n162 = call "Mapping Simulated Spectrum v10.6.4.vi"() -> ("Simulated Spectrum"=w328:cluster{i32[], dbl[]}[])
                                }
                                }
                                n163 = local read "Target Position"() -> (w292:T7)
                                n164 = Index Array(array=w286, index=0 ("Index")) -> (element=w285:T11)
                                n165 = call "Mapping Merge Live Data v10.2.1.vi"("New Spectrum"=w285, "Target Position"=w292, "X in (1D)"=w300, "Y in (1D)"=w299, "L in (2D)"=w298, "I in (2D)"=w297, "Step Size"=w283) -> ("Live Data"=w291:dbl[][], "X out (1D)"=w294:dbl[], "Y out (1D)"=w293:dbl[], "L out (2D)"=w295:dbl[][], "I out (2D)"=w296:dbl[][])  [unwired: 4 in]
                                n166 = invoke class="VI Interface Type 0" method="Ctrl Val.Set"(reference=w302, "Control Name"="LiveData" ("Elementname"), "Value"=w291) -> ()  [unwired: 2 in, 5 out]
                                n167 = local write "Live Data"(w291) -> ()
                              }
                            }
                          }
                          frame #4 {
                            # "set new X"
                            n168 = Increment(x=w339) -> (x+1=w338:i32)
                            n169 = local read "Start"() -> (w332:bool)
                            n170 = Equal?(x=w337, y=w338) -> (x = y?=w329:bool)
                            n171 = Not(x=w332) -> (.not. x?=w331:bool)
                            n172 = Or(x=w329, y=w331) -> (x .or. y?=w330:bool)
                            n173 = case shown="False" w330 {
                              tunnel: w336 -> [w347 w355]
                              tunnel: [w346 w355] -> w333
                              tunnel: w335 -> [w345 _]
                              tunnel: w334 -> [w340 _]
                              frame False {
                                n174 = Unbundle By Name(w347) -> ("Drive X Position"=w348:dbl)
                                n175 = case shown="False" w345 {
                                tunnel: w348 -> [w351 w353]
                                tunnel: [w350 w354] -> w341
                                tunnel: w340 -> [w349 w352]
                                frame False {
                                n176 = Subtract(x=w351, y=w349) -> (x-y=w350:dbl)
                                }
                                frame True {
                                n177 = Add(x=w353, y=w352) -> (x+y=w354:dbl)
                                }
                                }
                                n178 = Divide(x=w341, y=w340) -> (x/y=w344:dbl)
                                n179 = Round To Nearest(number=w344) -> (nearest integer value=w343:dbl)
                                n180 = Multiply(x=w343, y=w340) -> (x*y=w342:dbl)
                                n181 = Bundle By Name(cluster=w347, "Drive X Position"=w342) -> (w346:T3)
                              }
                              frame True {
                              }
                            }
                            n182 = local write "Target Position"(w333) -> ()
                          }
                          frame #5 {
                            n183 = Tick Count (ms)() -> (millisecond timer value=w360:u32)
                            n184 = Subtract(x=w360, y=w359) -> (x-y=w362:u32)
                            n185 = Divide(x=w362, y=u32 1000) -> (x/y=w357:dbl)
                            n186 = Build Array (concatenate)(w358, w357) -> (w356:dbl[])
                          }
                          frame #6 {
                            # "update countdown"
                            n187 = Array Size(array=w368) -> (size(s)=w367:i32[])
                            n188 = local read "Mapping Params"() -> (w372:T8)
                            n189 = Index Array(array=w367, index=0) -> (element=w364:i32)
                            n190 = Increment "The data array is not\nyet updated with the\ncurrent run."(x=w364) -> (x+1=w363:i32)
                            n191 = call "Mapping Countdown v10.6.3.vi"("Execution Times (s)"=w369, "Mapping Spectra Settings"=w370, "Ready Steps"=w363, "Mapping Drive Parameters"=w372) -> ("Progress"=→"Progress":i16, "Time String"=w371:string)  [unwired: 6 in]
                            n192 = property on="Measuring" class="Bool (strict)"("BoolText.Text"=w371) -> ()  [unwired: 2 in, 2 out]
                          }
                        }
                        n193 = local read "Start"() -> (w221:bool)
                      }
                    }
                    frame #1 {
                      # "autosave current map"
                      n194 = local read "AutoSave Inc."() -> (w374:i16)
                      n195 = local read "Progress"() -> (w377:u8)
                      n196 = Quotient & Remainder(x=w377, y=w374) -> (floor(x/y)=w379:i16)  [unwired: 1 out]
                      n197 = Quotient & Remainder(x=w380, y=w374) -> (floor(x/y)=w378:i16)  [unwired: 1 out]
                      n198 = Greater?(x=w379, y=w378) -> (0:w376:bool)
                      n199 = Greater Than 0?(x=w374) -> (x > 0?=w375:bool)
                      n200 = And(x=w376, y=w375) -> (x .and. y?=w373:bool)
                      n201 = case shown="True" w373 {
                        tunnel: w383 -> [_ w391]
                        tunnel: w382 -> [_ w390]
                        tunnel: [w384 w387] -> w381
                        tunnel: w380 -> [w384 _]
                        tunnel: w377 -> [_ w387]
                        frame False {
                        }
                        frame True {
                          n202 = local read "Input Parameters"() -> (w404:T1)
                          n203 = global read "Global Variables.vi" "Global iHR Values"() -> (w401:T4)
                          n204 = global read "Global Variables.vi" "Global ITC Values"() -> (w400:T2)
                          n205 = local read "Spectra Params"() -> (w403:T5)
                          n206 = global read "Global Variables.vi" "Global CCD Temperature (C)"() -> (w402:dbl)
                          n207 = Unbundle By Name(w404) -> ("CCD Area"=w405:T6, "CCD Gain"=w407:u16, "CCD ADC"=w406:u16)
                          n208 = Number To Fractional String(number=w387, precision (6)=i16 0) -> (F-format string=w385:string)  [unwired: 2 in]
                          n209 = local read "Mapping Params"() -> (w408:T8)
                          n210 = global read "Global Variables.vi" "Mapping Autosave Folder"() -> (w388:path)
                          n211 = call "Export_mappingFileName v10.5.1.vi"("ITC503 Current Values"=w400, "iHR Current Values"=w401, "Spectra Settings"=w403, "Mapping Parameters"=w408) -> ("Filename"=w395:string)  [unwired: 1 in]
                          n212 = local read "Live Data"() -> (w397:dbl[][])
                          n213 = Unbundle By Name(w408) -> ("Step Size"=w399:dbl)
                          n214 = call "Mapping Merge Real Positions v10.2.1.vi"("Live Data In"=w397, "X in (1D)"=w391, "Y in (1D)"=w390, "Step Size"=w399) -> ("Live Data Out"=w398:dbl[][])  [unwired: 11 in]
                          n215 = Concatenate Strings(w395, "_" ("string"), w385, "pct" ("string")) -> (w392:string)
                          n216 = call "Export_2DtoTxt v10.6.3.vi"("ITC503 Current Values"=w400, "iHR Current Values"=w401, "CCD Temperature"=w402, "CCD Area"=w405, "CCD ADC"=w406, "CCD Gain"=w407, "Auto?"=TRUE, "Export Type"="Mapping", "Spectra Settings"=w403, "Filename"=w392, "Data (2D)"=w398, "Auto Folder"=w388, "Mapping Parameters"=w408) -> ()  [unwired: 6 in, 1 out]
                        }
                      }
                    }
                    frame #2 {
                      # "set new Y and move\nto new position"
                      n217 = Increment(x=w421) -> (x+1=w420:i32)
                      n218 = local read "Start"() -> (w411:bool)
                      n219 = Equal?(x=w419, y=w420) -> (x = y?=w413:bool)
                      n220 = Not(x=w411) -> (.not. x?=w412:bool)
                      n221 = Or(x=w413, y=w412) -> (x .or. y?=w410:bool)
                      n222 = case shown="False" w410 {
                        tunnel: w417 -> [w444 w445]
                        tunnel: [w443 w445] -> w415
                        tunnel: w418 -> [w437 _]
                        frame False {
                          n223 = Unbundle By Name(w444) -> ("Drive Y Position"=w438:dbl)
                          n224 = Add(x=w438, y=w437) -> (x+y=w440:dbl)
                          n225 = Divide(x=w440, y=w437) -> (x/y=w441:dbl)
                          n226 = Round To Nearest(number=w441) -> (nearest integer value=w442:dbl)
                          n227 = Multiply(x=w442, y=w437) -> (x*y=w439:dbl)
                          n228 = Bundle By Name(cluster=w444, "Drive Y Position"=w439) -> (w443:T3)
                        }
                        frame True {
                        }
                      }
                      n229 = local read "Simulate Drive"() -> (w414:bool)
                      n230 = case shown="False" w414 {
                        tunnel: w416 -> [w426 _]
                        tunnel: w415 -> [w425 _]
                        tunnel: w409 -> [w423 _]
                        frame False {
                          n231 = flat-sequence {
                            tunnel: w426 -> [w432]
                            tunnel: w425 -> [w431]
                            tunnel: [w432] -> w427
                            tunnel: w423 -> [w428]
                            tunnel: [w428] -> w422
                            tunnel: [w436] -> w424
                            tunnel: w427 -> [w435]
                            tunnel: w422 -> [w434]
                            frame #0 {
                              n232 = Unbundle By Name(w431) -> ("Drive Y Position"=w430:dbl)
                              n233 = control-ref of="Objective Running"() -> (w433:refnum<vi>)
                              n234 = call "NPC3SG Move Axis To v10.6.2.vi"("Drive Visa Name"=w432, "Running"=w433, "Axis"=1, "Drive Set"=w430, "Calibration File"=w428) -> ()  [unwired: 2 in, 1 out]
                            }
                            frame #1 {
                              n235 = call "NPC3SG Get Positions v10.6.2.vi"("Drive Visa Name"=w435, "Calibration File"=w434) -> ("Drive Current Values"=w436:T3)  [unwired: 5 in]
                            }
                          }
                          n236 = global write "Global Variables.vi" "Global Piezo Position"(w424) -> ()
                          n237 = local write "Current Position"(w424) -> ()
                        }
                        frame True {
                        }
                      }
                      n238 = local write "Target Position"(w415) -> ()
                    }
                  }
                  n239 = local read "Start"() -> (w162:bool)
                }
              }
              frame #2 {
                # "conclude measurement"
                n240 = flat-sequence {
                  tunnel: w447 -> [w460]
                  tunnel: w446 -> [w459]
                  tunnel: w448 -> [w465]
                  frame #0 {
                    # "save data"
                    n241 = local read "Input Parameters"() -> (w453:T1)
                    n242 = global read "Global Variables.vi" "Global iHR Values"() -> (w456:T4)
                    n243 = global read "Global Variables.vi" "Global ITC Values"() -> (w457:T2)
                    n244 = local read "Spectra Params"() -> (w454:T5)
                    n245 = global read "Global Variables.vi" "Global CCD Temperature (C)"() -> (w455:dbl)
                    n246 = Unbundle By Name(w453) -> ("CCD Area"=w452:T6, "CCD Gain"=w450:u16, "CCD ADC"=w451:u16)
                    n247 = local read "Mapping Params"() -> (w449:T8)
                    n248 = call "Export_mappingFileName v10.5.1.vi"("ITC503 Current Values"=w457, "iHR Current Values"=w456, "Spectra Settings"=w454, "Mapping Parameters"=w449) -> ("Filename"=w463:string)  [unwired: 1 in]
                    "Filename" <- w463
                    n249 = local read "Live Data"() -> (w462:dbl[][])
                    n250 = Unbundle By Name(w449) -> ("Step Size"=w458:dbl)
                    n251 = call "Mapping Merge Real Positions v10.2.1.vi"("Live Data In"=w462, "X in (1D)"=w460, "Y in (1D)"=w459, "Step Size"=w458) -> ("Live Data Out"=w461:dbl[][])  [unwired: 11 in]
                    "Full Data" <- w461
                    n252 = call "Export_2DtoTxt v10.6.3.vi"("ITC503 Current Values"=w457, "iHR Current Values"=w456, "CCD Temperature"=w455, "CCD Area"=w452, "CCD ADC"=w451, "CCD Gain"=w450, "Export Type"="Mapping", "Spectra Settings"=w454, "Filename"=w463, "Data (2D)"=w461, "Mapping Parameters"=w449) -> ()  [unwired: 8 in, 1 out]
                  }
                  frame #1 {
                    # "reset indicators"
                    n253 = local write "Start"(FALSE ("Start")) -> ()
                    n254 = local write "CCD Current Rep."("0/0" ("CCD3000 Current Rep.")) -> ()
                    n255 = case shown="False" w465 {
                      frame False {
                        n256 = call "Video Toolset Stop.vi"() -> ()  [unwired: 3 in]
                      }
                      frame True {
                      }
                    }
                    n257 = property on="Measuring" class="Bool (strict)"("BoolText.Text"="" ("Boolescher Text.Text")) -> ()  [unwired: 2 in, 2 out]
                    n258 = property on="Measuring" class="Bool (strict)"("Blinking"=FALSE ("Measuring")) -> ()  [unwired: 2 in, 2 out]
                    n259 = global write "Global Variables.vi" "Mapping Running?"(FALSE ("Mapping Running?")) -> ()
                  }
                }
              }
            }
          }
        }
        n260 = local read "Exit"() -> (w47:bool)
      }
    }
    frame #2 {
      n261 = invoke class="VI Interface Type 0" method="Ctrl Val.Set"(reference=w472, "Control Name"="Exit" ("Elementname"), "Value"=TRUE) -> ()  [unwired: 2 in, 5 out]
      n262 = local read "AutoClose"() -> (w471:bool)
      n263 = flat-sequence {
        tunnel: w471 -> [w475]
        frame #0 {
          # "reset and close"
          n264 = control-ref of="Dieses VI"() -> (w478:refnum<vi>)
          n265 = global write "Global Variables.vi" "Mapping Open?"(FALSE ("Mapping Open?")) -> ()
          n266 = invoke class="VI" method="Default Vals.Reinit All"(reference=w478) -> (reference out=w476:refnum<vi>)  [unwired: 2 in, 2 out]
          n267 = property on="Measuring" class="Bool (strict)"("BoolText.Text"="" ("Boolescher Text.Text")) -> ()  [unwired: 2 in, 2 out]
          n268 = property class="App"() -> ("App.Kind"=w479:T12)  [unwired: 2 in, 2 out]
          n269 = case shown="\"invalid app kind\", Default" w479 {
            tunnel: w476 -> [w481 w483]
            tunnel: w475 -> [_ w482]
            frame "invalid app kind", Default {
              n270 = invoke on="Invoke Node" class="VI" method="FP.Close"(reference=w481) -> ()  [unwired: 2 in, 3 out]
            }
            frame "Development System" {
              n271 = case shown="True" w482 {
                tunnel: w483 -> [_ w484]
                frame False {
                }
                frame True {
                  n272 = invoke on="Invoke Node" class="VI" method="FP.Close"(reference=w484) -> ()  [unwired: 2 in, 3 out]
                }
              }
            }
          }
        }
      }
    }
  }
